vi "multi_plots_cluster.vi"() -> ()   [LabVIEW 2022 SP3]
panel:
  out "Waveform Graph":cluster{dbl[]}[](graph)
  out "Waveform Chart":cluster{dbl, dbl}[](graph)
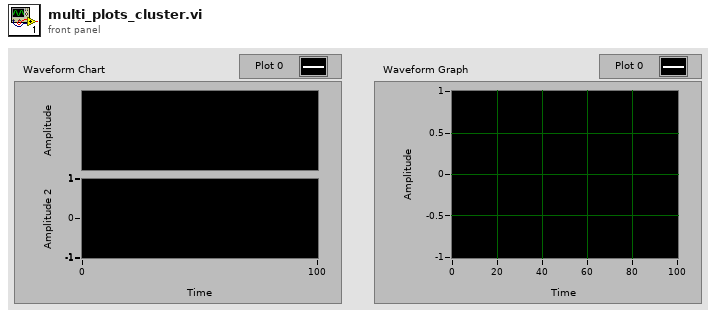
[diagram p1: front panel]
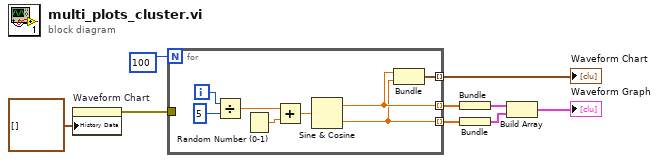
[diagram p0: block diagram]
diagram:
  n1 = property on="Waveform Chart" class="WFChart (严格)"("History Data"=cluster{dbl, dbl}[] []) -> (error out=w8:errorcluster)  [unwired: 2 in, 1 out]
  n2 = for {
    N: 100 -> [_]
    tunnel: w8 -> [_]
    tunnel: [w12] -> w7 mode=indexing
    tunnel: [w11] -> w5 mode=indexing
    tunnel: [w10] -> w4 mode=indexing
    i -> [w17]
    n3 = Divide(x=w17, y=5) -> (x/y=w14:dbl)
    n4 = Random Number (0-1)() -> (number: 0 to 1=w15:dbl)
    n5 = Add(x=w14, y=w15) -> (x+y=w13:dbl)
    n6 = Sine & Cosine(0:w13) -> (1:w11:dbl, 2:w10:dbl)
    n7 = Bundle "Bundle"(w11, w10) -> (w12:cluster{dbl, dbl})  [unwired: 1 in]
  }
  "Waveform Chart" <- w7
  n8 = Bundle "Bundle"(w5) -> (w3:cluster{dbl[]})  [unwired: 1 in]
  n9 = Bundle(w4) -> (w2:cluster{dbl[]})  [unwired: 1 in]
  n10 = Build Array "Build Array"(w3, w2) -> (→"Waveform Graph":cluster{dbl[]}[])
